vi "Find Local Chassis.vi"(8 "error in":errorcluster, 11 "scan engine custom device ref in":T1 format="%.0x") -> (0 "error out":errorcluster, 1 "slots refs":T1[](array[typedef]) format="%.0x", 2 "local chassis ref":T1 format="%.0x", 3 "scan engine custom device ref out":T1 format="%.0x", 4 "user variables ref":T1=18446744073709551615 format="%.0x", 5 "found":bool)   [LabVIEW 2020, in "Scan Engine Scripting.lvlib"]
doc: "Returns the local chassis found in the Scan Engine and EtherCAT custom device."
uses:
  Scan Engine Scripting.lvlib
  <vilib>/NI VeriStand/Custom Device API/Custom Device Item Ref.ctl
  Scan Engine Dependencies.llb/Scan Engine GUIDs.vi
  <vilib>/NI VeriStand/Custom Device Tools/Custom Device Utility Library/NI VeriStand - Search for Item by GUID.vi
  Utility/Ref Constants.vi
  Scan Engine Dependencies.llb/Scan Engine Custom Device.lvlib
  <vilib>/NI VeriStand/Custom Device Tools/Custom Device Utility Library/Custom Device Utility Library.lvlib
  <vilib>/NI VeriStand/Custom Device API/Custom Device API.lvlib
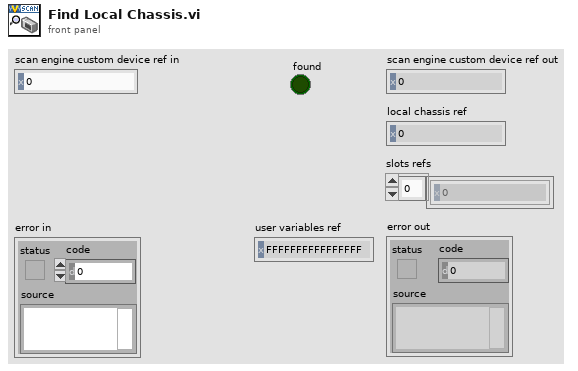
[diagram p1: front panel]
types:
  T1 = typedef "Custom Device API.lvlib/Custom Device Item Ref.ctl" = u64
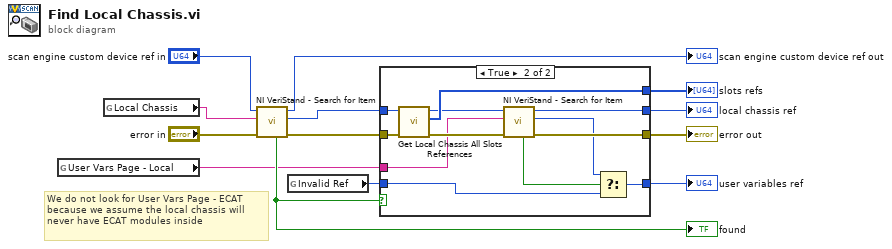
[diagram p0: block diagram]
diagram:
  # "We do not look for User Vars Page - ECAT because we assume the local chassis will never have ECAT modules inside"
  n1 = global read "Scan Engine GUIDs.vi" "User Vars Page - Local"() -> (w1:string)
  n2 = global read "Scan Engine GUIDs.vi" "Local Chassis"() -> (w10:string)
  n3 = call-poly <vilib>:"NI VeriStand - Search for Item.vi"("error in"="error in", "Item GUID"=w10, "Section Ref in"="scan engine custom device ref in") -> ("error out"=w8:errorcluster, "Item Ref"=w7:T1, "Section Ref out"=→"scan engine custom device ref out":T1, "Found"=w4:bool)  [unwired: 5 in]
  "found" <- w4
  n4 = global read "Ref Constants.vi" "Invalid Ref"() -> (w2:T1)
  n5 = case shown="True" w4 {
    tunnel: [w16 w24] -> w9
    tunnel: w8 -> [w16 w28]
    tunnel: w7 -> [w15 w27]
    tunnel: [w15 w22] -> w6
    tunnel: [_ w26] -> w5
    tunnel: w1 -> [_ w21]
    tunnel: [w14 w18] -> w3
    tunnel: w2 -> [w14 w17]
    frame False {
      # "Did not find a local chassis"
    }
    frame True {
      n6 = call "Get Local Chassis All Slots References.vi"("error in"=w28, "Local Chassis Reference In"=w27) -> ("error out"=w25:errorcluster, "Slots References"=w26:T1[], "Local Chassis Reference Out"=w23:T1)  [unwired: 6 in, 1 out]
      n7 = call-poly <vilib>:"NI VeriStand - Search for Item.vi"("error in"=w25, "Item GUID"=w21, "Section Ref in"=w23) -> ("error out"=w24:errorcluster, "Item Ref"=w19:T1, "Section Ref out"=w22:T1, "Found"=w20:bool)  [unwired: 5 in]
      n8 = Select(t=w19, s=w20, f=w17) -> (s? t:f=w18:T1)
    }
  }
  "error out" <- w9
  "local chassis ref" <- w6
  "slots refs" <- w5
  "user variables ref" <- w3
